vi "DequeueElement.vi"(11 "queue":string) -> (3 "element":string)   [LabVIEW 2011]
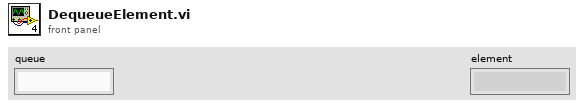
[diagram p1: front panel]
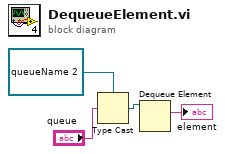
[diagram p0: block diagram]
diagram:
  n1 = Type Cast(type=refnum<queue> refnum ("队列输出"), x="queue") -> (*(type *) &x=w2:refnum<queue>)
  n2 = Dequeue Element(queue=w2) -> (element=→"element":string)  [unwired: 2 in, 3 out]
